vi "Cross Power Spectrum PtByPt.vi"(4 "initialize":bool, 5 "dt":dbl=1.0 format="%0.2f", 6 "sample length":i32=100, 7 "signal y":dbl format="%0.2f", 8 "signal x":dbl format="%0.2f") -> (0 "error":i32, 1 "df":dbl format="%0.2f", 2 "Cross Power XY Spectrum Phase (radians)":dbl[](array[numeric]), 3 "Cross Power XY Spectrum Mag (V^2rms)":dbl[](array[numeric]))   [LabVIEW 2020, in "NI_PtbyPt.lvlib"]
doc: "Computes the single-sided, scaled, cross power spectrum of two real-time signals."
uses:
  <vilib>/ptbypt/NI_PtbyPt.lvlib
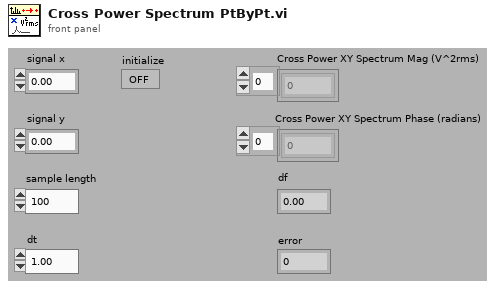
[diagram p1: front panel]
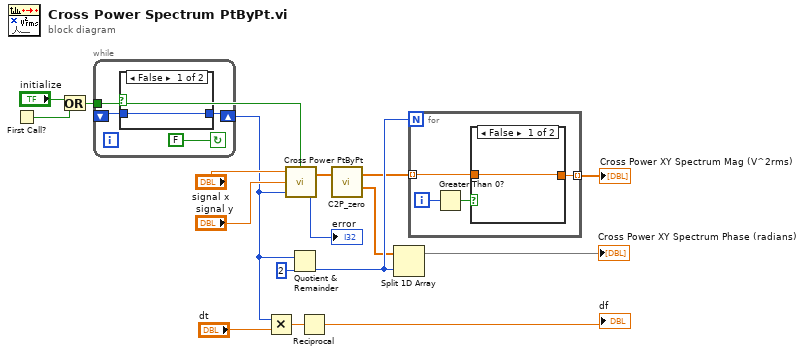
[diagram p0: block diagram]
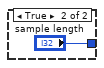
[diagram p2: hidden frame]
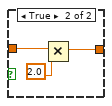
[diagram p3: hidden frame]
diagram:
  n1 = First Call?() -> (First Call?: T/F=w3:bool)
  n2 = Or(x="initialize", y=w3) -> (x .or. y?=w2:bool)
  n3 = while {
    tunnel: w2 -> [w19]
    shift-left: _ -> [w20]
    shift-right: [w21] -> w1
    stop <- FALSE continue-if-true
    n4 = case shown="False" w19 {
      tunnel: [w22 "sample length"] -> w21
      tunnel: w20 -> [w22 _]
      frame False {
      }
      frame True {
      }
    }
  }
  n5 = Multiply(x=w1, y="dt") -> (x*y=w17:dbl)
  n6 = call <vilib>:"Cross Power PtByPt.vi"("initialize"=w2, "sample length"=w1, "y"="signal y", "x"="signal x") -> ("error"=→"error":i32, "Sxy"=w6:cdb[])
  n7 = Quotient & Remainder(x=w1, y=2) -> (floor(x/y)=w9:i32)  [unwired: 1 out]
  n8 = Reciprocal(x=w17) -> (1/x=→"df":dbl)
  n9 = call <vilib>:"C2P_zero.vi"("r * e^(i*theta)"=w6) -> ("amplitude"=w5:dbl[], "phase"=w4:dbl[])
  n10 = Split 1D Array(array=w4, index=w9) -> (first subarray=→"Cross Power XY Spectrum Phase (radians)":dbl[])  [unwired: 1 out]
  n11 = for {
    N: w9 -> [_]
    tunnel: [w25] -> w13 mode=indexing
    tunnel: w5 -> [w24] mode=indexing
    i -> [w27]
    n12 = Greater Than 0?(x=w27) -> (x > 0?=w26:bool)
    n13 = case shown="False" w26 {
      tunnel: [w28 w31] -> w25
      tunnel: w24 -> [w28 w30]
      frame False {
      }
      frame True {
        n14 = Multiply(x=w30, y=2.0) -> (x*y=w31:dbl)
      }
    }
  }
  "Cross Power XY Spectrum Mag (V^2rms)" <- w13
